vi "Configure IP Setup.vi"(0 "VISA resource name":refnum<visa-resource-name>, 5 "IP Setup Mode (0:Auto)":u16(ring) items=["Auto", "Manual"], 11 "error in (no error)":errorcluster) -> (4 "VISA resource name out":refnum<visa-resource-name>, 15 "error out":errorcluster)   [LabVIEW 2014, in "eec EST 300.lvlib"]
doc: "Sets the IP Setup Mode Of the APT 6000 Series Power Source instrument\n\nThe Ethernet card is set to Auto configure the IP address through DHCP. \nIf the user changes to Manual configuration they must set the IP address manually."
uses:
  <instrlib>/eec EST 300/eec EST 300.lvlib
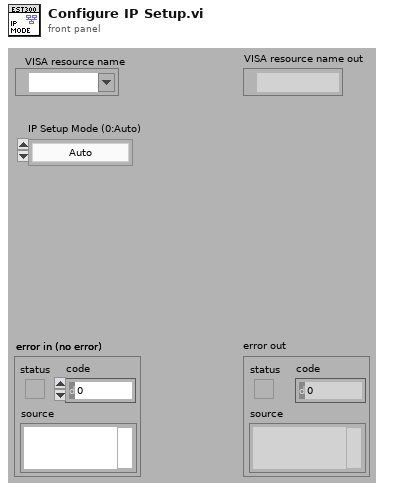
[diagram p1: front panel]
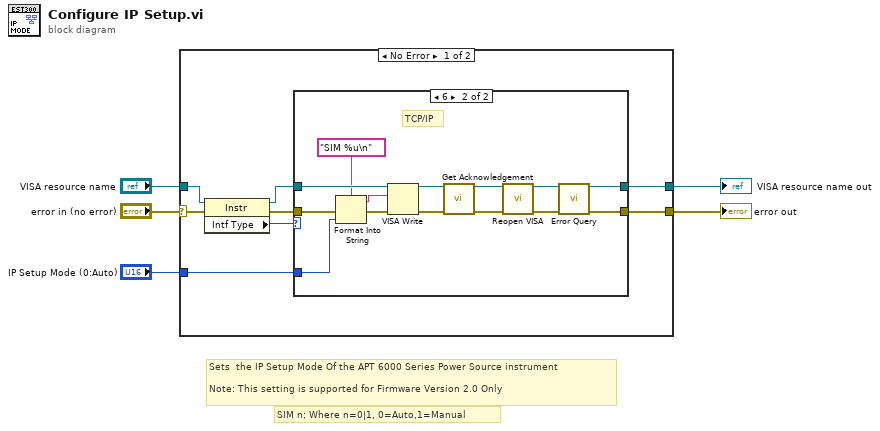
[diagram p0: block diagram]
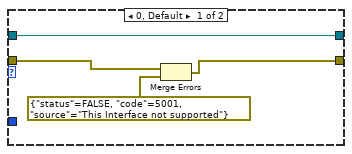
[diagram p2: hidden frame]
diagram:
  # "SIM n; Where n=0|1, 0=Auto,1=Manual"
  # "Sets  the IP Setup Mode Of the APT 6000 Series Power Source instrument\n\nNote: This setting is supported for Firmware Version 2.0 Only"
  n1 = case shown="No Error" "error in (no error)" {
    selector: "error in (no error)" -> [w11 w33]
    tunnel: "VISA resource name" -> [w8 w32]
    tunnel: [w13 w32] -> w5
    tunnel: [w12 w33] -> w4
    tunnel: "IP Setup Mode (0:Auto)" -> [w10 _]
    frame No Error {
      n2 = property class="Instr"(reference=w8, error in=w11) -> (reference out=w7:refnum<visa-resource-name>, error out=w9:errorcluster, "Intf Type"=w6:u16)
      n3 = case shown="6" w6 {
        tunnel: w7 -> [w17 w31]
        tunnel: [w17 w30] -> w13
        tunnel: [w14 w28] -> w12
        tunnel: w9 -> [w15 w26]
        tunnel: w10 -> [_ w23]
        frame 0, Default {
          n4 = Merge Errors(w15, errorcluster {"status"=FALSE, "code"=5001, "source"="This Interface not supported"} ("error in 2 (no error)")) -> (w14:errorcluster)
        }
        frame 6 {
          # "TCP/IP"
          n5 = Format Into String(format string="SIM %u\n" ("Command to Send"), error in=w26, w23) -> (resulting string=w27:string, error out=w25:errorcluster)  [unwired: 1 in]
          n6 = VISA Write(VISA resource name=w31, write buffer=w27, error in (no error)=w25) -> (VISA resource name out=w21:refnum<visa-resource-name>, error out=w29:errorcluster)  [unwired: 1 out]
          n7 = call <instrlib>:"Get Acknowledgement.vi"("VISA resource name"=w21, "error in (no error)"=w29) -> ("VISA resource name out"=w19:refnum<visa-resource-name>, "error out"=w22:errorcluster)  [unwired: 12 in]
          n8 = call <instrlib>:"Reopen VISA.vi"("VISA resource name"=w19, "error in (no error)"=w22) -> ("VISA resource name out"=w18:refnum<visa-resource-name>, "error out"=w20:errorcluster)  [unwired: 12 in]
          n9 = call <instrlib>:"Error Query.vi"("VISA resource name"=w18, "error in (no error)"=w20) -> ("VISA resource name out"=w30:refnum<visa-resource-name>, "error out"=w28:errorcluster)  [unwired: 10 in, 2 out]
        }
      }
    }
    frame Error {
    }
  }
  "error out" <- w4
  "VISA resource name out" <- w5
